vi "wrap.LoadBuffer.vi"(0 "class.GLue in":refnum<class "class.GLue.lvclass">, 2 "Script":string, 11 "error in (no error)":errorcluster, 13 "ChunkName":string) -> (4 "class.GLue out":refnum<class "class.GLue.lvclass">, 6 "Error":string, 10 "return type":i32, 15 "error out":errorcluster)   [LabVIEW 2014, in "GLue.lvlib" / "class.GLue.lvclass"]
uses:
  class.GLue.lvclass
  class.GLue.lvclass/class.GLue.ctl
  Resources/GLue.dll
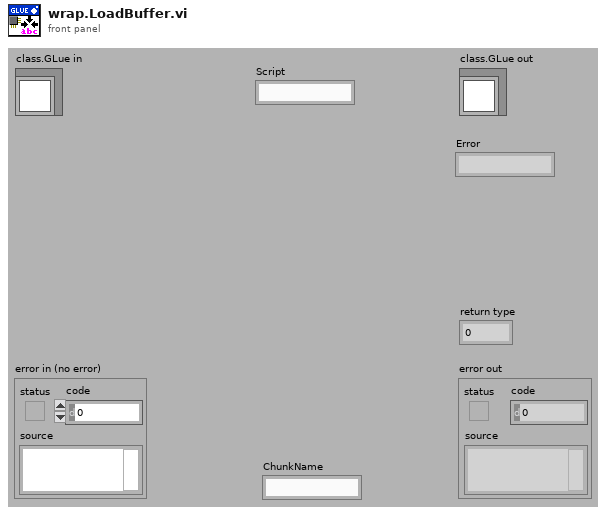
[diagram p1: front panel]
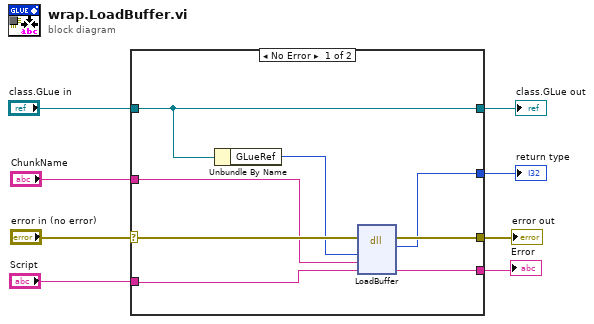
[diagram p0: block diagram]
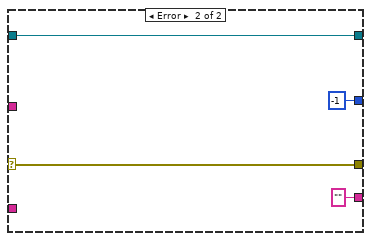
[diagram p2: hidden frame]
diagram:
  n1 = case shown="No Error" "error in (no error)" {
    selector: "error in (no error)" -> [w15 w20]
    tunnel: [w14 w20] -> w7
    tunnel: [w16 w19] -> w5
    tunnel: "class.GLue in" -> [w16 w19]
    tunnel: "ChunkName" -> [w12 _]
    tunnel: [w11 -1 ("return type")] -> w3
    tunnel: [w10 "" ("Error")] -> w2
    tunnel: "Script" -> [w9 _]
    frame No Error {
      n2 = Unbundle By Name(w16) -> ("GLueRef"=w13:i64)
      n3 = dll-call lib="C:/Users/Antonie/Documents/work/glue/trunk/Resources/GLue.dll" fn="LoadBuffer"(error in=w15, "GLue"=w13, "ChunkName"=w12, "ScriptString"=w9) -> (error out=w14:errorcluster, "return type"=w11:i32, "ScriptString"=w10:string)  [unwired: 4 in, 1 out]
    }
    frame Error {
    }
  }
  "error out" <- w7
  "class.GLue out" <- w5
  "return type" <- w3
  "Error" <- w2
